vi "GOOPUtil_FindAllGOOPKernels.vi"(0 "AllApplications":bool, 1 "ClassNames":string[](array[string]), 5 "error in (no error)":errorcluster) -> (15 "GOOPKernels":T1[](array[typedef]), 19 "error out":errorcluster)   [LabVIEW 2014, in "GOOPUtility.lvlib"]
doc: "Finds all GOOP kernals in all application instances and return information about them in the selected list. If the class name list is empty, all GOOP Kernels in memory will be returned."
uses:
  <vilib>/addons/GOOPUtility/GOOPUtility.lvlib
  <vilib>/Utility/allVIsInMemory.llb/VIMemory VI info.ctl
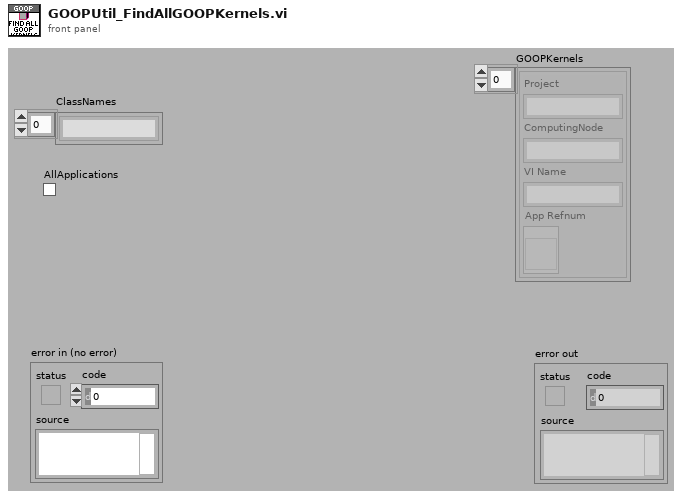
[diagram p1: front panel]
types:
  T1 = typedef "VIMemory VI info.ctl" = cluster{"Project":string, "ComputingNode":string, "VI Name":string, "App Refnum":refnum<vi>}
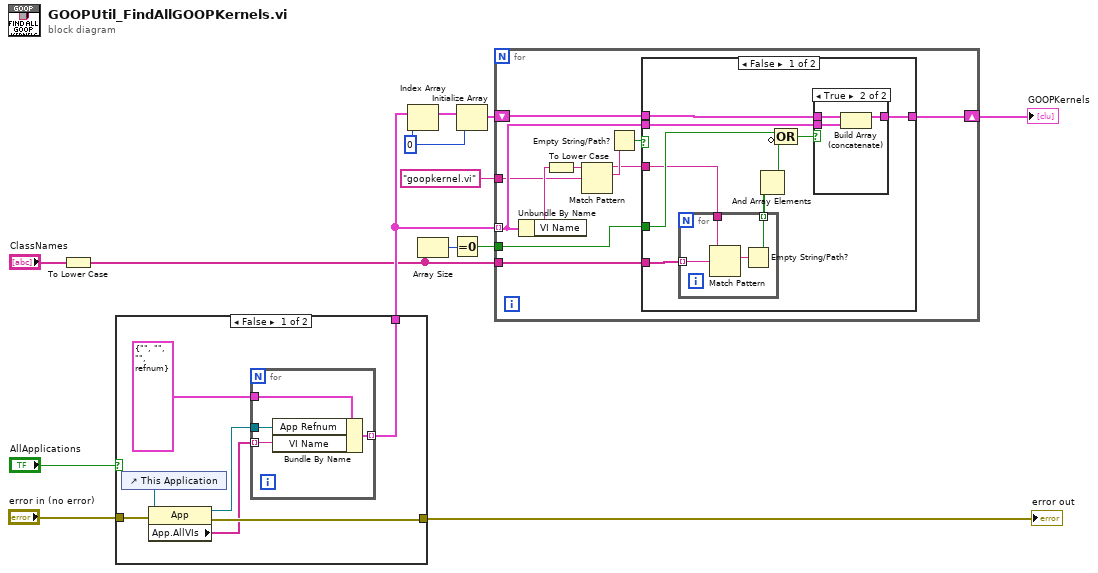
[diagram p0: block diagram]
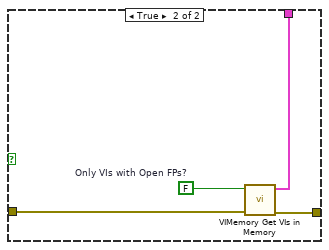
[diagram p2: hidden frame]
diagram:
  w10 = 0 ("index")
  n1 = To Lower Case(string="ClassNames") -> (all lower case string=w4:string[])
  n2 = case shown="False" "AllApplications" {
    tunnel: [w14 w27] -> w13
    tunnel: [w18 w25] -> w1
    tunnel: "error in (no error)" -> [w20 w26]
    frame False {
      n3 = control-ref of="This Application"() -> (w19:refnum<vi>)
      n4 = property class="App"(reference=w19, error in=w20) -> (reference out=w15:refnum<vi>, error out=w18:errorcluster, "App.AllVIs"=w16:string[])
      n5 = for {
        tunnel: T1 {"Project"="", "ComputingNode"="", "VI Name"="", "App Refnum"=refnum} ("VI info") -> [w24]
        tunnel: w16 -> [w23] mode=indexing
        tunnel: w15 -> [w22]
        tunnel: [w21] -> w14 mode=indexing
        n6 = Bundle By Name(cluster=w24, "App Refnum"=w22, "VI Name"=w23) -> (w21:T1)
      }
    }
    frame True {
      w28 = FALSE  # Only VIs with Open FPs?
      n7 = call <vilib>:"VIMemory Get VIs in Memory.vi"("error in (no error)"=w26, "Only VIs with Open FPs?"=w28) -> ("error out"=w25:errorcluster, "VIs in memory"=w27:T1[])  [unwired: 8 in]
    }
  }
  "error out" <- w1
  n8 = Index Array(array=w13, index=w10) -> (element=w11:T1)
  n9 = Array Size(array=w4) -> (size(s)=w6:i32)
  n10 = Equal To 0?(x=w6) -> (x = 0?=w5:bool)
  n11 = Initialize Array(w11, w10) -> (w12:T1[])
  n12 = for {
    tunnel: w13 -> [w38] mode=indexing
    shift-right: [w37] -> w8
    shift-left: w12 -> [w39]
    tunnel: "goopkernel.vi" -> [w34]
    tunnel: w4 -> [w31]
    tunnel: w5 -> [w30]
    n13 = Unbundle By Name(w38) -> ("VI Name"=w36:string)
    n14 = To Lower Case(string=w36) -> (all lower case string=w35:string)
    n15 = Match Pattern(string=w35, regular expression=w34) -> (before substring=w29:string, match substring=w33:string)  [unwired: 1 in, 2 out]
    n16 = Empty String/Path?(string/path=w33) -> (empty?=w32:bool)
    n17 = case shown="False" w32 {
      tunnel: w39 -> [w48 w57]
      tunnel: w38 -> [w47 _]
      tunnel: [w46 w57] -> w37
      tunnel: w31 -> [w43 _]
      tunnel: w30 -> [w45 _]
      tunnel: w29 -> [w42 _]
      frame False {
        n18 = for {
          tunnel: w43 -> [w52] mode=indexing
          tunnel: w42 -> [w51]
          tunnel: [w49] -> w41 mode=indexing
          n19 = Match Pattern(string=w51, regular expression=w52) -> (match substring=w50:string)  [unwired: 1 in, 3 out]
          n20 = Empty String/Path?(string/path=w50) -> (empty?=w49:bool)
        }
        n21 = And Array Elements(Boolean array=w41) -> (logical AND=w40:bool)
        n22 = Compound Arithmetic op=OR(w45, invert w40) -> (w44:bool)
        n23 = case shown="True" w44 {
          tunnel: w48 -> [w53 w56]
          tunnel: w47 -> [_ w55]
          tunnel: [w53 w54] -> w46
          frame False {
          }
          frame True {
            n24 = Build Array (concatenate)(w56, w55) -> (w54:T1[])
          }
        }
      }
      frame True {
      }
    }
  }
  "GOOPKernels" <- w8
